vi "关键参数交互.vi"(9 "量程下拉列表":refnum<vi>, 10 "测量模式下拉列表":refnum<vi>, 11 "参数下拉列表":refnum<vi>) -> ()   [LabVIEW 2016, in "斯坦道氨氮.lvlib"]
panel:
  out "x != y?":T1
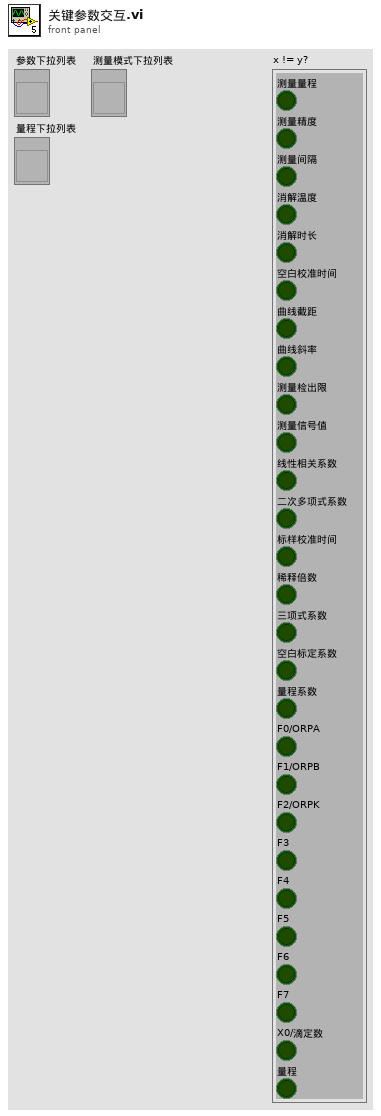
[diagram p1: front panel]
types:
  T1 = cluster{"测量量程":bool, "测量精度":bool, "测量间隔":bool, "消解温度":bool, "消解时长":bool, "空白校准时间":bool, "曲线截距":bool, "曲线斜率":bool, "测量检出限":bool, "测量信号值":bool, "线性相关系数":bool, "二次多项式系数":bool, "标样校准时间":bool, "稀释倍数":bool, "三项式系数":bool, "空白标定系数":bool, "量程系数":bool, "F0/ORPA":bool, "F1/ORPB":bool, "F2/ORPK":bool, "F3":bool, "F4":bool, "F5":bool, "F6":bool, "F7":bool, "X0/滴定数":bool, "量程":bool}
  T2 = cluster{"chose":string, "公式":cluster{"X^2":dbl, "X":dbl, "b":dbl}}
  T3 = cluster{"测量量程":dbl, "测量精度":dbl, "测量间隔":dbl, "消解温度":dbl, "消解时长":dbl, "空白校准时间":timestamp, "曲线截距":dbl, "曲线斜率":dbl, "测量检出限":dbl, "测量信号值":dbl, "线性相关系数":dbl, "二次多项式系数":dbl, "标样校准时间":timestamp, "稀释倍数":dbl, "三项式系数":dbl, "空白标定系数":dbl, "量程系数":dbl, "F0/ORPA":dbl, "F1/ORPB":dbl, "F2/ORPK":dbl, "F3":dbl, "F4":dbl, "F5":dbl, "F6":dbl, "F7":dbl, "X0/滴定数":dbl, "量程":dbl}
  T4 = cluster{"时间标识":timestamp, "设备":string, "日志信息":string, "流程参数":string}
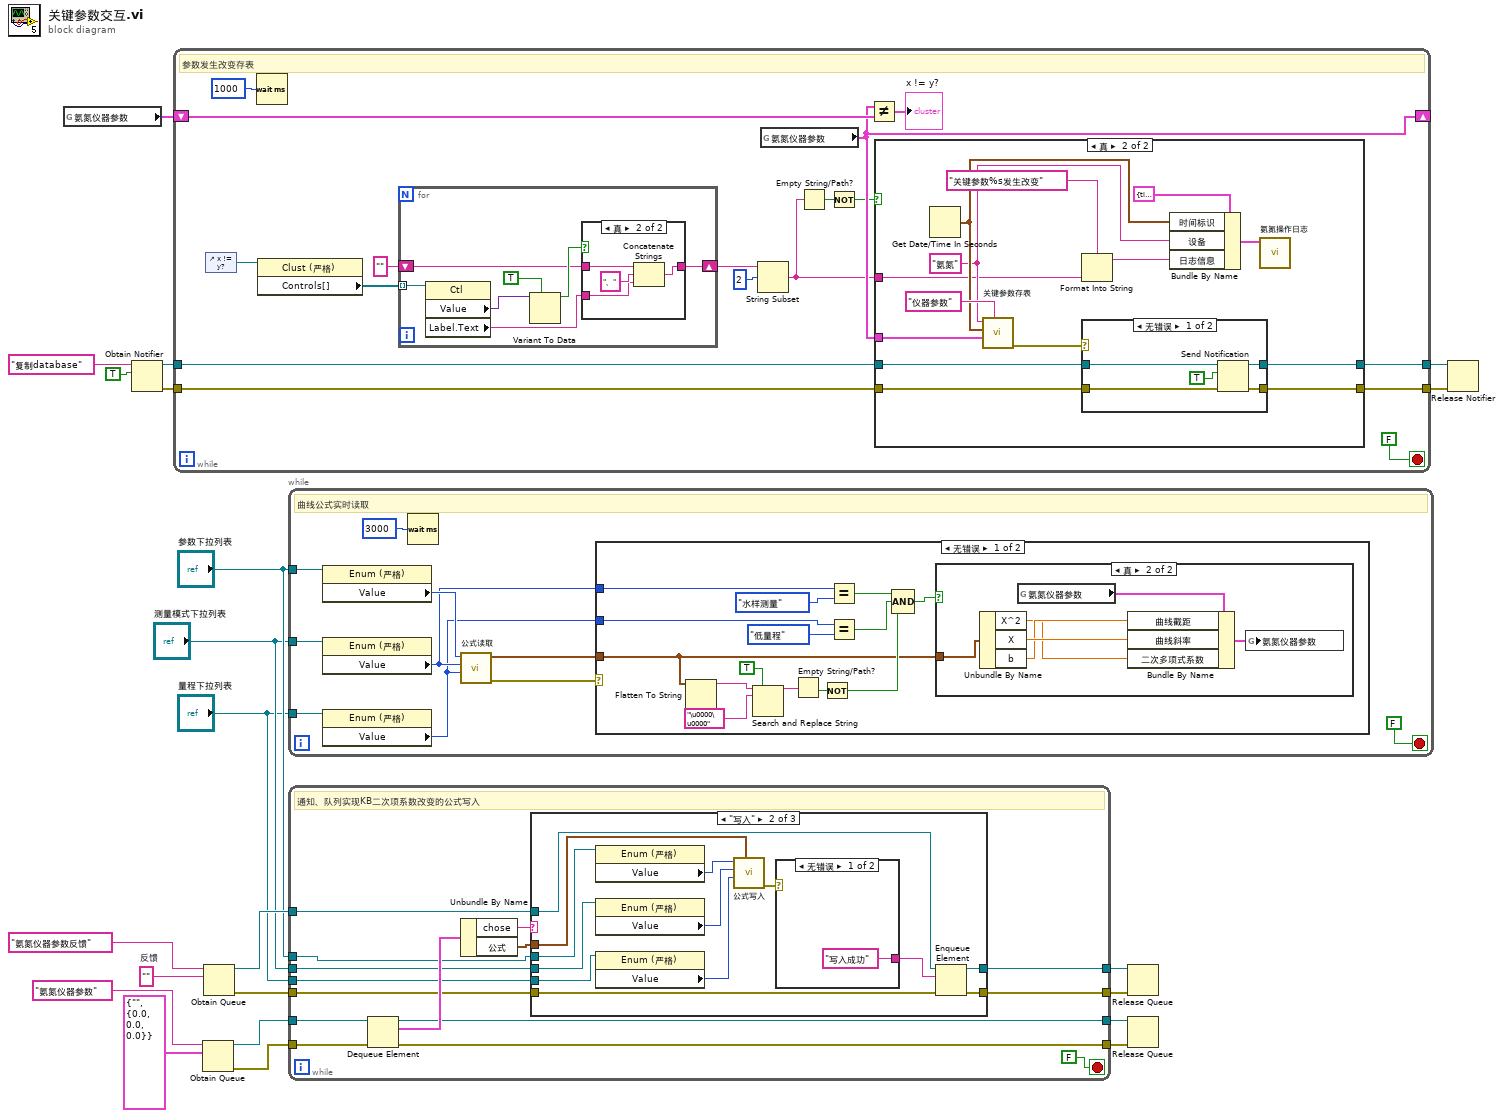
[diagram p0: block diagram]
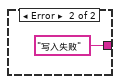
[diagram p5: hidden frame]
diagram:
  w15 = ""  # 反馈
  n1 = global read "氨氮断电保存全局变量.vi" "氨氮仪器参数"() -> (w22:T3)
  n2 = Obtain Notifier(name (unnamed)="复制database" ("名称（未命名）"), notification data type=TRUE) -> (notifier out=w4:refnum<notifier>, error out=w3:errorcluster)  [unwired: 2 in, 1 out]
  n3 = while {
    shift-right: [w34] -> _
    shift-left: w22 -> [w37]
    tunnel: w4 -> [w33]
    tunnel: w3 -> [w32]
    tunnel: [w31] -> w2
    tunnel: [w30] -> w1
    stop <- FALSE stop-if-true
    # "参数发生改变存表"
    n4 = control-ref of="x != y?"() -> (w35:refnum<vi>)
    n5 = Wait (ms)(milliseconds to wait=u32 1000 ("等待时间（毫秒）")) -> ()  [unwired: 1 out]
    n6 = property class="Clust (严格)"(reference=w35) -> ("Controls[]"=w26:refnum<vi>[])  [unwired: 1 in, 2 out]
    n7 = for {
      tunnel: w26 -> [w46] mode=indexing
      shift-right: [w40] -> w28
      shift-left: "" -> [w42]
      n8 = property class="Ctl"(reference=w46) -> ("Value"=w44:variant, "Label.Text"=w41:string)  [unwired: 1 in, 2 out]
      n9 = Variant To Data(type=TRUE, Variant=w44) -> (data=w43:bool)  [unwired: 1 in, 1 out]
      n10 = case shown="真" w43 {
        tunnel: w42 -> [w47 w51]
        tunnel: w41 -> [_ w48]
        tunnel: [w47 w50] -> w40
        frame False {
        }
        frame True {
          n11 = Concatenate Strings(w51, "、", w48) -> (w50:string)
        }
      }
    }
    n12 = String Subset(string=w28, offset (0)=2 ("偏移量(0)")) -> (substring=w23:string)  [unwired: 1 in]
    n13 = global read "氨氮断电保存全局变量.vi" "氨氮仪器参数"() -> (w34:T3)
    n14 = Empty String/Path?(string/path=w23) -> (empty?=w25:bool)
    n15 = Not(x=w25) -> (.not. x?=w24:bool)
    n16 = Not Equal?(x=w34, y=w37) -> (x != y?=→"x != y?":T1)
    n17 = case shown="真" w24 {
      tunnel: w34 -> [_ w66]
      tunnel: w23 -> [_ w60]
      tunnel: w33 -> [w53 w58]
      tunnel: w32 -> [w52 w57]
      tunnel: [w53 w55] -> w31
      tunnel: [w52 w54] -> w30
      frame False {
      }
      frame True {
        w62 = "氨氮" ("仪器名称")
        n18 = Get Date/Time In Seconds() -> (seconds since 1Jan1904=w63:timestamp)
        n19 = call "关键参数存表.vi"("table"="仪器参数", "仪器参数"=w66, "datatime"=w63, "仪器名称"=w62) -> ("error out"=w56:errorcluster)  [unwired: 7 in]
        n20 = Format Into String(format string="关键参数%s发生改变" ("格式字符串"), w60) -> (resulting string=w59:string)  [unwired: 2 in, 1 out]
        n21 = case shown="无错误" w56 {
          tunnel: w58 -> [w72 w74]
          tunnel: w57 -> [w71 w73]
          tunnel: [w69 w74] -> w55
          tunnel: [w68 w73] -> w54
          frame No Error {
            n22 = Send Notification(notification=TRUE ("通知"), notifier=w72, error in (no error)=w71) -> (notifier out=w69:refnum<notifier>, error out=w68:errorcluster)
          }
          frame Error {
          }
        }
        n23 = Bundle By Name(cluster=T4 {"时间标识"=timestamp(0 s since 1904-01-01), "设备"="", "日志信息"="", "流程参数"=""} ("data in"), "时间标识"=w63, "设备"=w62, "日志信息"=w59) -> (w64:T4)
        n24 = call "氨氮操作日志.vi"("data in"=w64) -> ()  [unwired: 11 in]
      }
    }
  }
  n25 = Obtain Queue(name (unnamed)="氨氮仪器参数" ("名称（未命名）"), element data type=T2 {"chose"="", "公式"={"X^2"=0.0, "X"=0.0, "b"=0.0}}) -> (queue out=w11:refnum<queue>, error out=w10:errorcluster)  [unwired: 3 in, 1 out]
  n26 = Obtain Queue(name (unnamed)="氨氮仪器参数反馈" ("名称（未命名）"), element data type=w15) -> (queue out=w16:refnum<queue>, error out=w14:errorcluster)  [unwired: 3 in, 1 out]
  n27 = while {
    tunnel: "参数下拉列表" -> [w77]
    tunnel: "测量模式下拉列表" -> [w76]
    tunnel: "量程下拉列表" -> [w75]
    stop <- FALSE stop-if-true
    # "曲线公式实时读取"
    n28 = property class="Enum (严格)"(reference=w77) -> ("Value"=w82:enum16{"总磷", "总氮", "氨氮"})  [unwired: 1 in, 2 out]
    n29 = property class="Enum (严格)"(reference=w76) -> ("Value"=w80:enum16{"水样测量", "零点核查", "跨度核查", "标样核查", "加标回收"})  [unwired: 1 in, 2 out]
    n30 = property class="Enum (严格)"(reference=w75) -> ("Value"=w79:enum16{"低量程", "高量程"})  [unwired: 1 in, 2 out]
    n31 = Wait (ms)(milliseconds to wait=u32 3000 ("等待时间（毫秒）")) -> ()  [unwired: 1 out]
    n32 = call "公式读取.vi"("量程"=w79, "测量模式"=w80, "测量参数"=w82) -> ("error out"=w78:errorcluster, "公式"=w81:cluster{"X^2":dbl, "X":dbl, "b":dbl})  [unwired: 7 in]
    n33 = case shown="无错误" w78 {
      tunnel: w80 -> [w98 _]
      tunnel: w81 -> [w85 _]
      tunnel: w79 -> [w92 _]
      frame No Error {
        n34 = Flatten To String(anything=w85) -> (data string=w91:string)  [unwired: 3 in, 2 out]
        n35 = Search and Replace String(replace all?=TRUE ("替换全部？(F)"), input string=w91, search string="\u0000\u0000" ("数据字符串")) -> (result string=w90:string)  [unwired: 5 in, 3 out]
        n36 = Empty String/Path?(string/path=w90) -> (empty?=w89:bool)
        n37 = Not(x=w89) -> (.not. x?=w86:bool)
        n38 = Equal?(x=w98, y=enum16{"水样测量", "零点核查", "跨度核查", "标样核查", "加标回收"}."水样测量") -> (x = y?=w95:bool)
        n39 = Equal?(x=w92, y=enum16{"低量程", "高量程"}."低量程") -> (x = y?=w94:bool)
        n40 = Compound Arithmetic op=AND ("复合运算")(w95, w94, w86) -> (w93:bool)
        n41 = case shown="真" w93 {
          tunnel: w85 -> [_ w102]
          frame False {
          }
          frame True {
            n42 = Unbundle By Name(w102) -> ("X^2"=w99:dbl, "X"=w101:dbl, "b"=w100:dbl)
            n43 = global read "氨氮断电保存全局变量.vi" "氨氮仪器参数"() -> (w104:T3)
            n44 = Bundle By Name(cluster=w104, "曲线截距"=w100, "曲线斜率"=w101, "二次多项式系数"=w99) -> (w103:T3)
            n45 = global write "氨氮断电保存全局变量.vi" "氨氮仪器参数"(w103) -> ()
          }
        }
      }
      frame Error {
      }
    }
  }
  n46 = while {
    tunnel: w11 -> [w118]
    tunnel: w10 -> [w117]
    tunnel: [w109] -> w19
    tunnel: [w108] -> w18
    tunnel: w16 -> [w113]
    tunnel: w14 -> [w112]
    tunnel: [w111] -> w13
    tunnel: [w110] -> w12
    tunnel: "参数下拉列表" -> [w107]
    tunnel: "测量模式下拉列表" -> [w106]
    tunnel: "量程下拉列表" -> [w105]
    stop <- FALSE stop-if-true
    # "通知、队列实现KB二次项系数改变的公式写入"
    n47 = Dequeue Element(queue=w118, error in (no error)=w117) -> (queue out=w109:refnum<queue>, element=w116:T2, error out=w108:errorcluster)  [unwired: 1 in, 1 out]
    n48 = Unbundle By Name(w116) -> ("chose"=w115:string, "公式"=w114:cluster{"X^2":dbl, "X":dbl, "b":dbl})
    n49 = case shown="\"写入\"" w115 {
      tunnel: w114 -> [_ w130 _]
      tunnel: w113 -> [w121 w129 w138]
      tunnel: w112 -> [w120 w127 w137]
      tunnel: [w121 w126 w138] -> w111
      tunnel: [w120 w125 w137] -> w110
      tunnel: w107 -> [_ w124 _]
      tunnel: w106 -> [_ w123 _]
      tunnel: w105 -> [_ w122 _]
      frame "假", Default {
      }
      frame "写入" {
        n50 = property class="Enum (严格)"(reference=w124) -> ("Value"=w132:enum16{"总磷", "总氮", "氨氮"})  [unwired: 1 in, 2 out]
        n51 = property class="Enum (严格)"(reference=w123) -> ("Value"=w133:enum16{"水样测量", "零点核查", "跨度核查", "标样核查", "加标回收"})  [unwired: 1 in, 2 out]
        n52 = property class="Enum (严格)"(reference=w122) -> ("Value"=w134:enum16{"低量程", "高量程"})  [unwired: 1 in, 2 out]
        n53 = call "公式写入.vi"("公式"=w130, "量程"=w134, "测量模式"=w133, "测量参数"=w132) -> ("error out"=w131:errorcluster)  [unwired: 7 in]
        n54 = case shown="无错误" w131 {
          tunnel: ["写入成功" ("消息") "写入失败" ("消息")] -> w128
          frame No Error {
          }
          frame Error {
          }
        }
        n55 = Enqueue Element(queue=w129, element=w128, error in (no error)=w127) -> (queue out=w126:refnum<queue>, error out=w125:errorcluster)  [unwired: 1 in, 1 out]
      }
      frame "读取" {
      }
    }
  }
  n56 = Release Queue(queue=w13, error in (no error)=w12) -> ()  [unwired: 1 in, 3 out]
  n57 = Release Queue(queue=w19, error in (no error)=w18) -> ()  [unwired: 1 in, 3 out]
  n58 = Release Notifier(notifier=w2, error in (no error)=w1) -> ()  [unwired: 1 in, 3 out]
